vi "pid_tanh.vi"(0 "err":dbl, 1 "kp":dbl, 2 "kd":dbl, 3 "ki":dbl, 5 "d_err":dbl, 7 "i_error":dbl, 12 "max_u":dbl) -> (15 "u":dbl)   [LabVIEW 2019]
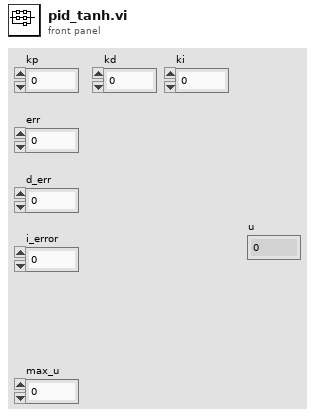
[diagram p1: front panel]
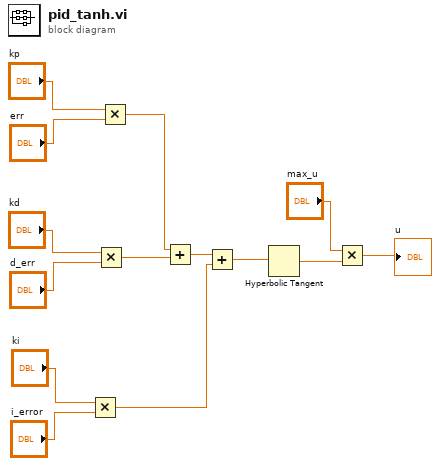
[diagram p0: block diagram]
diagram:
  n1 = Multiply(x="ki", y="i_error") -> (x*y=w5:dbl)
  n2 = Multiply(x="kd", y="d_err") -> (x*y=w8:dbl)
  n3 = Multiply(x="kp", y="err") -> (x*y=w6:dbl)
  n4 = Add(x=w6, y=w8) -> (x+y=w7:dbl)
  n5 = Add(x=w7, y=w5) -> (x+y=w4:dbl)
  n6 = Hyperbolic Tangent(1:w4) -> (0:w3:dbl)
  n7 = Multiply(x="max_u", y=w3) -> (x*y=→"u":dbl)
